vi "DefenderAreaRoleVSS.vi"(7 "First call?":bool=TRUE, 8 "error in (no error)":errorcluster, 9 "Game in":refnum<class "Game.lvclass">, 11 "DefenderAreaRoleVSS in":refnum<class "DefenderAreaRoleVSS.lvclass">) -> (0 "error out":errorcluster, 1 "Game out":refnum<class "Game.lvclass">, 2 "Robot out":refnum<class "Robot.lvclass">, 3 "DefenderAreaRoleVSS out":refnum<class "DefenderAreaRoleVSS.lvclass">)   [LabVIEW 2020, in "DefenderAreaRoleVSS.lvclass"]
uses:
  DefenderAreaRoleVSS.lvclass
  Robot_class/Robot.lvclass
  Game_class/Game.lvclass
  Role_class/Role.lvclass/Role.ctl
  Role_class/Read Tacticbook.vi
  Role_class/Read tactic_index.vi
  Role_class/Write Tacticbook.vi
  Role_class/Write tactic_index.vi
  Role_class/Read RobotRef.vi
  Tacticbook_class/Tacticbook.lvclass
  DispBallTacticVSS_class/DispBallTacticVSS.lvclass
  DefendGoalTacticVSS_class/DefendGoalTacticVSS.lvclass
  PenaltyAttackTacticVSS_class/PenaltyAttackTacticVSS.lvclass
  DefendAreaTacticVSS_class/DefendAreaTacticVSS.lvclass
  AttackTacticVSS_class/AttackTacticVSS.lvclass
  HaltTactic_class/HaltTactic.lvclass
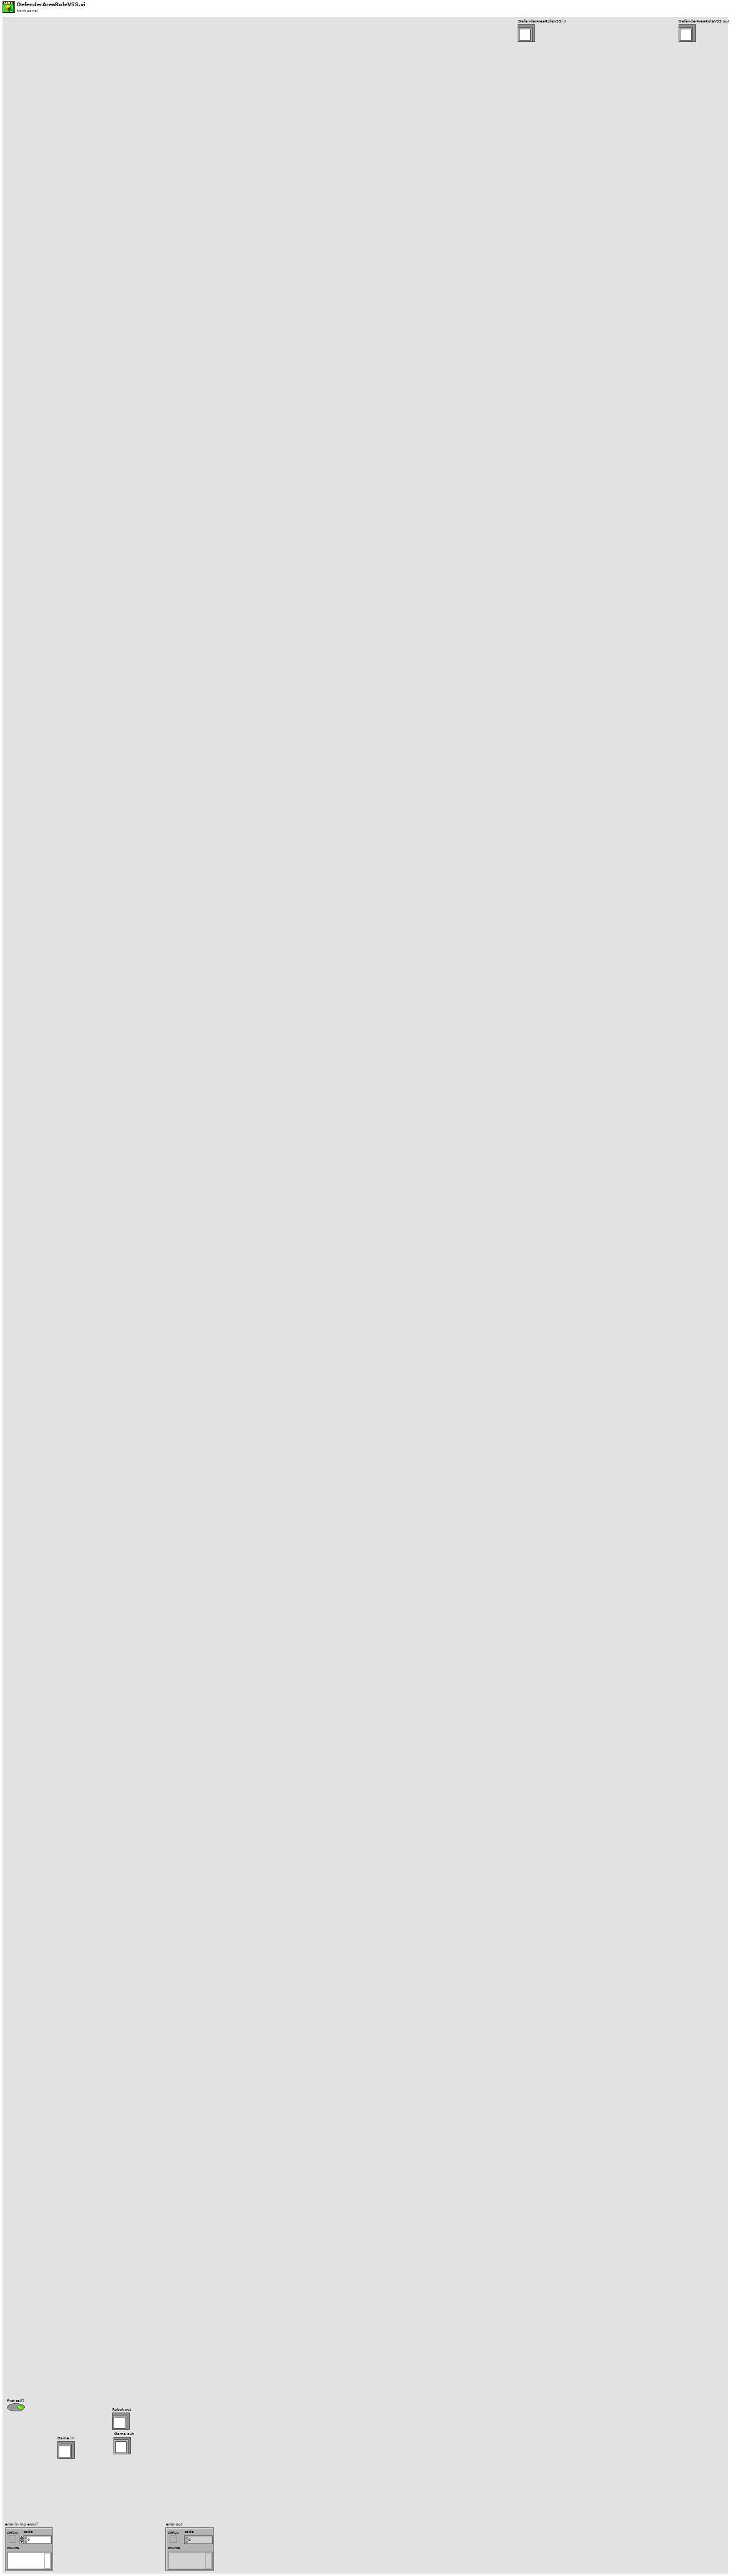
[diagram p1: front panel]
types:
  T1 = cluster{"DispBallTacticVSS":refnum<class "DispBallTacticVSS.lvclass">, "DefendGoalTacticVSS":refnum<class "DefendGoalTacticVSS.lvclass">, "PenaltyAttackTacticVSS":refnum<class "PenaltyAttackTacticVSS.lvclass">, "DefendAreaTacticVSS":refnum<class "DefendAreaTacticVSS.lvclass">, "AttackTacticVSS":refnum<class "AttackTacticVSS.lvclass">, "HaltTactic":refnum<class "HaltTactic.lvclass">}
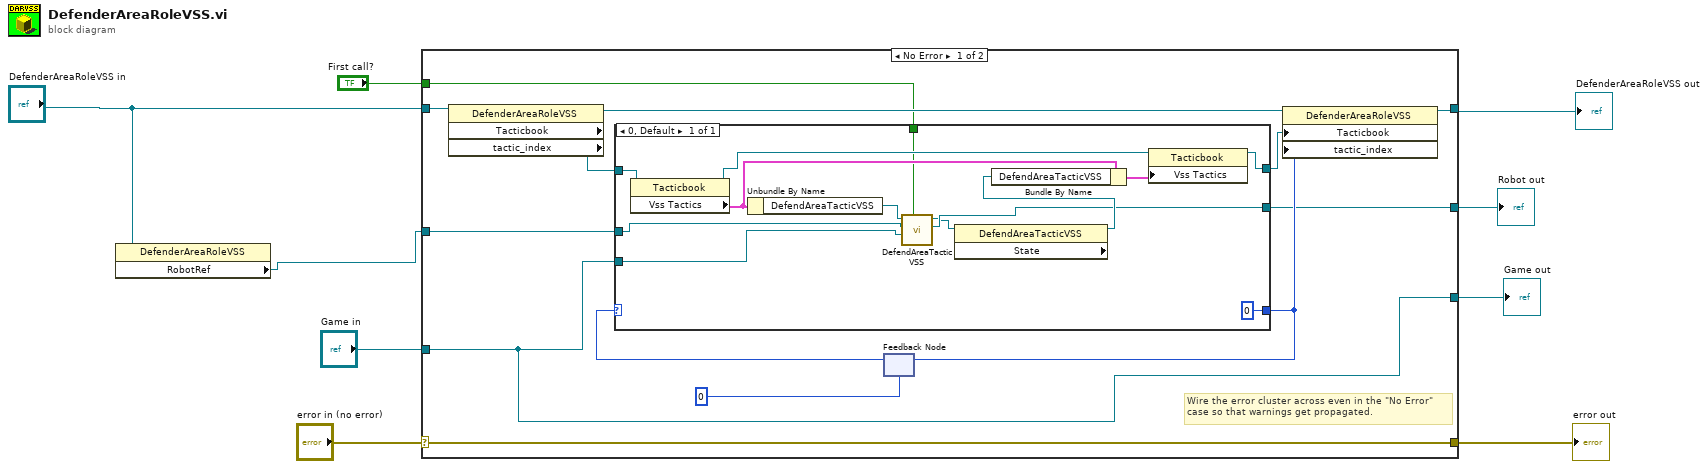
[diagram p0: block diagram]
diagram:
  n1 = property class="DefenderAreaRoleVSS"(reference="DefenderAreaRoleVSS in") -> ("RobotRef"=w3:refnum<class "Robot.lvclass">)  [unwired: 1 in, 2 out]
  n2 = case shown="No Error" "error in (no error)" {
    selector: "error in (no error)" -> [w22 w39]
    tunnel: [w22 w39] -> w8
    tunnel: [w20 w38] -> w2
    tunnel: "DefenderAreaRoleVSS in" -> [w21 w38]
    tunnel: w3 -> [w14 w37]
    tunnel: [w13 w37] -> w7
    tunnel: [w11 w36] -> w6
    tunnel: "Game in" -> [w11 w36]
    tunnel: "First call?" -> [w10 _]
    frame No Error {
      # "Wire the error cluster across even in the \"No Error\"\ncase so that warnings get propagated."
      n3 = property class="DefenderAreaRoleVSS" props=["Tacticbook", "tactic_index"](reference=w21) -> (reference out=w19:refnum<class "DefenderAreaRoleVSS.lvclass">, "Tacticbook"=w16:refnum<class "Tacticbook.lvclass">)  [unwired: 1 in, 2 out]
      n4 = feedback #1(0) -> (w17:i32)
      n5 = case shown="0, Default" w17 {
        tunnel: [0] -> w15
        tunnel: w16 -> [w35]
        tunnel: w14 -> [w24]
        tunnel: [w28] -> w13
        tunnel: [w33] -> w12
        tunnel: w11 -> [w23]
        tunnel: w10 -> [w26]
        frame 0, Default {
          n6 = property class="Tacticbook"(reference=w35) -> (reference out=w34:refnum<class "Tacticbook.lvclass">, "Vss Tactics"=w31:T1)  [unwired: 1 in, 1 out]
          n7 = Unbundle By Name(w31) -> ("DefendAreaTacticVSS"=w25:refnum<class "DefendAreaTacticVSS.lvclass">)
          n8 = call "DefendAreaTacticVSS.vi"("First call?"=w26, "Game in"=w23, "Robot"=w24, "DefendAreaTacticVSS in"=w25) -> ("Robot out"=w28:refnum<class "Robot.lvclass">, "DefendAreaTacticVSS out"=w27:refnum<class "DefendAreaTacticVSS.lvclass">)  [unwired: 5 in, 1 out]
          n9 = property class="DefendAreaTacticVSS" props=["State"](reference=w27) -> (reference out=w29:refnum<class "DefendAreaTacticVSS.lvclass">)  [unwired: 1 in, 2 out]
          n10 = Bundle By Name(cluster=w31, "DefendAreaTacticVSS"=w29) -> (w30:T1)
          n11 = property class="Tacticbook"(reference=w34, "Vss Tactics"=w30) -> (reference out=w33:refnum<class "Tacticbook.lvclass">)  [unwired: 1 in, 1 out]
        }
      }
      n12 = feedback-in #1(w15) -> ()
      n13 = property class="DefenderAreaRoleVSS"(reference=w19, "Tacticbook"=w12, "tactic_index"=w15) -> (reference out=w20:refnum<class "DefenderAreaRoleVSS.lvclass">)  [unwired: 1 in, 1 out]
    }
    frame Error {
    }
  }
  "DefenderAreaRoleVSS out" <- w2
  "error out" <- w8
  "Robot out" <- w7
  "Game out" <- w6
